vi "field emission sensor_v70.vi"() -> ()   [LabVIEW 2014]
uses:
  Keithley 24XX/Public/Data/Read (Single Point).vi
  Keithley 24XX/Keithley 24XX.lvlib
  <userlib>/Nanonis Prog Interface V5/Nanonis Prog Interface.lvlib
  <vilib>/Analysis/NI_AALBase.lvlib
panel:
  in  "Std threshold":dbl=5e-12 format="%#_6p"
  in  "Mean threshold":dbl=2e-11 format="%#_6p"
  out "ramp paused":bool
  out "x+y":sgl=1.4799449e-10
  out "amplitude":sgl(graph)=1.0739469e-11
  in  "Amplitude (V) (NaN=no change)":sgl=nan
  in  "Frequency (Hz) (NaN=no change)":sgl=nan format="%#_6p"
  in  "p Amplitude":dbl=-0.3 format="%#_6p"
  in  "amplitude max":sgl=1.5e-10 format="%#_6p"
  in  "Signal index (0-79)":i8=49
  out "amplitude":sgl=1.0739469e-11 format="%#_6p"
  in  "dz":dbl=1e-09 format="%#_6p"
  in  "ramp delay (s)":dbl=0.001
  out "ramp trigger":bool
  out "millisecond timer value":u32=272952714
  in  "Clear plots":bool
  out "z":dbl(graph)=7.783200430924225e-08
  in  "Ramp":bool
  in  "steps":sgl=5e-09 format="%#_6p"
  in  "Ramp to":sgl=1.3e-06 format="%#_6p"
  in  "I":sgl=5e-05 format="%#_6p"
  in  "PID":bool
  in  "p":sgl=0.01 format="%#_6p"
  in  "setpoint":sgl format="%#_3p"
  in  "max Current":sgl=2e-06 format="%#_6p"
  in  "setpoint approach":sgl=3e-08 format="%#_6p"
  in  "auto approach":bool
  in  "Number of steps":u16=1
  in  "withdraw tip":bool
  in  "coarse step":bool
  in  "Direction":enum16{"X +", "X -", "Y +", "Y -", "Z +", "Z -"}(ring)=enum."Z +"
  in  "Machine name (local machine IP)":string="localhost"
  in  "Z position [m]":dbl=7.783200430924225e-08 max=1.096e-07 step=1.0 format="%_6p"
  out "current [A]":sgl=-1.479945e-08 format="%#_6p"
  in  "time divider":dbl=60.0
  out "time elapsed":dbl=72.48559594154358
  in  "milliseconds to wait":u32=100
  in  "VISA resource name":refnum<visa-resource-name>="GPIB0::21::INSTR"
  in  "stop":bool
  in  "current multiplier":sgl=1.0
  out "Current":sgl(graph)=-1.479945e-08
  # "STOP the VI during an Nanonis Auto Approach"
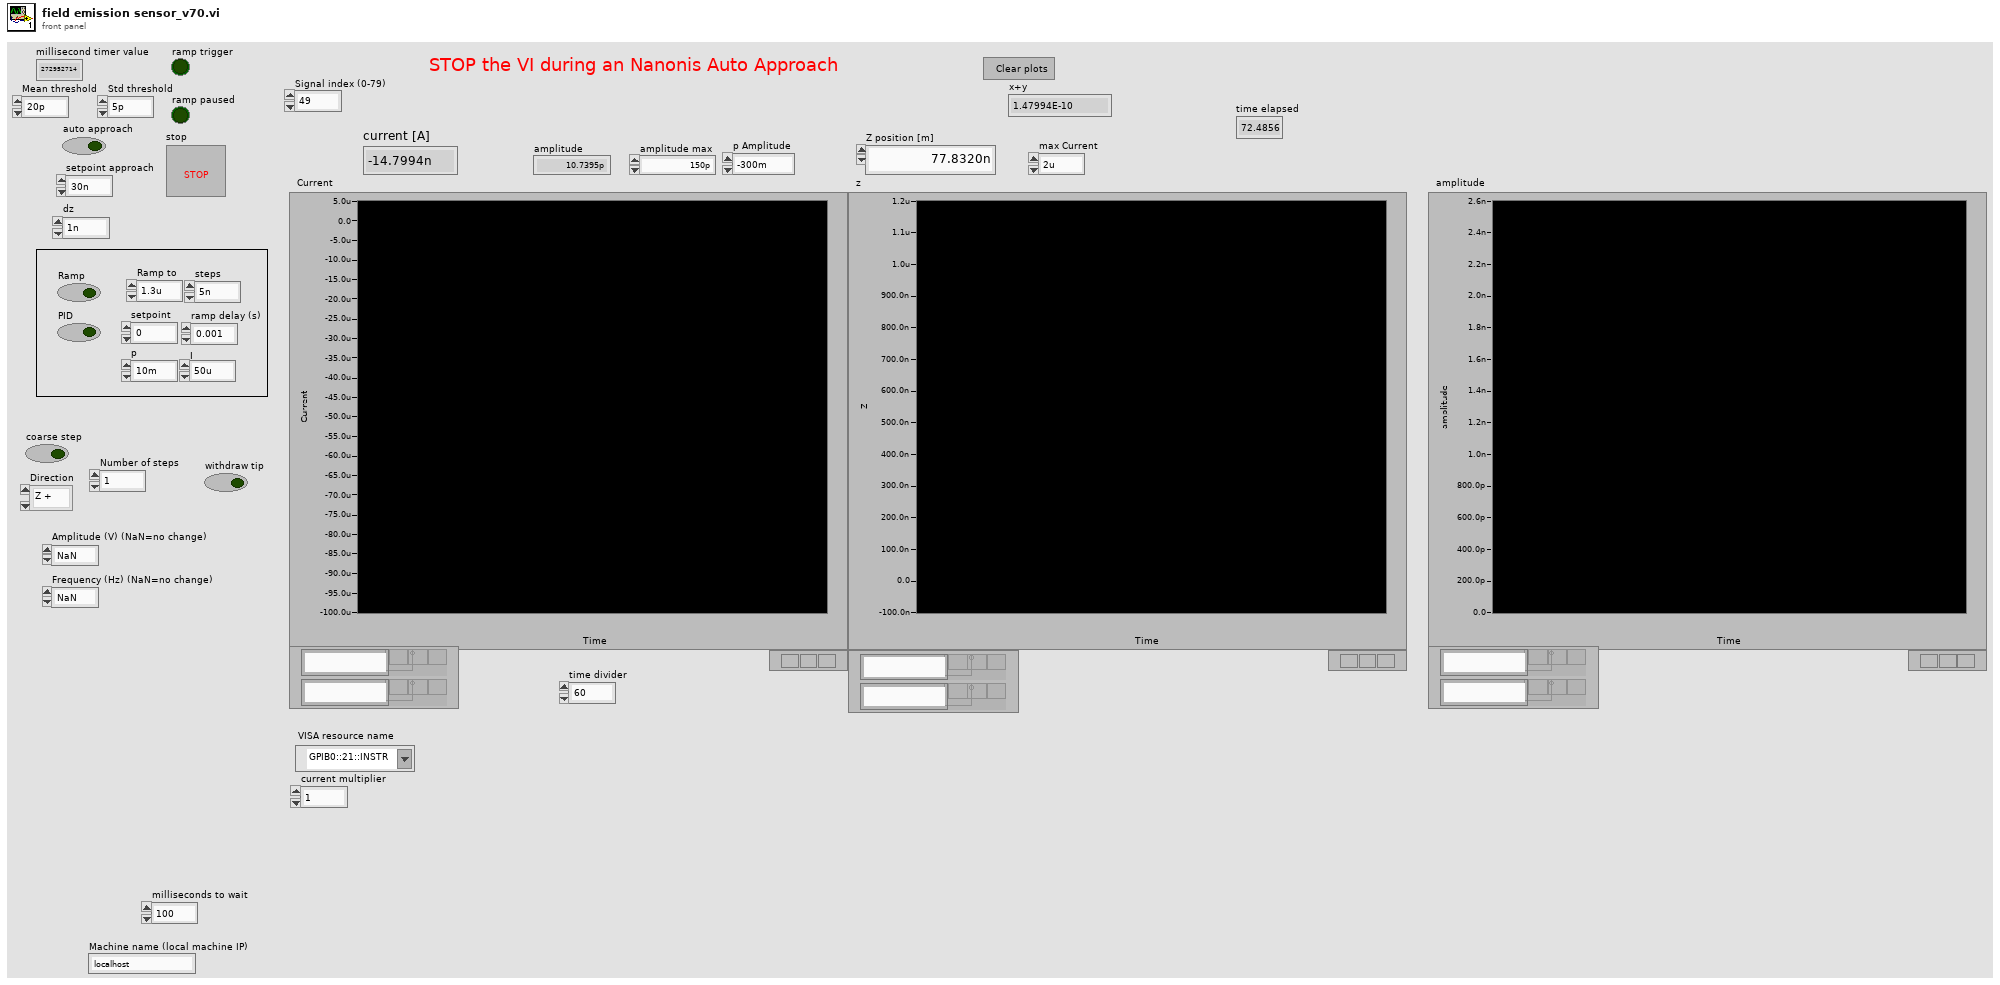
[diagram p1: front panel]
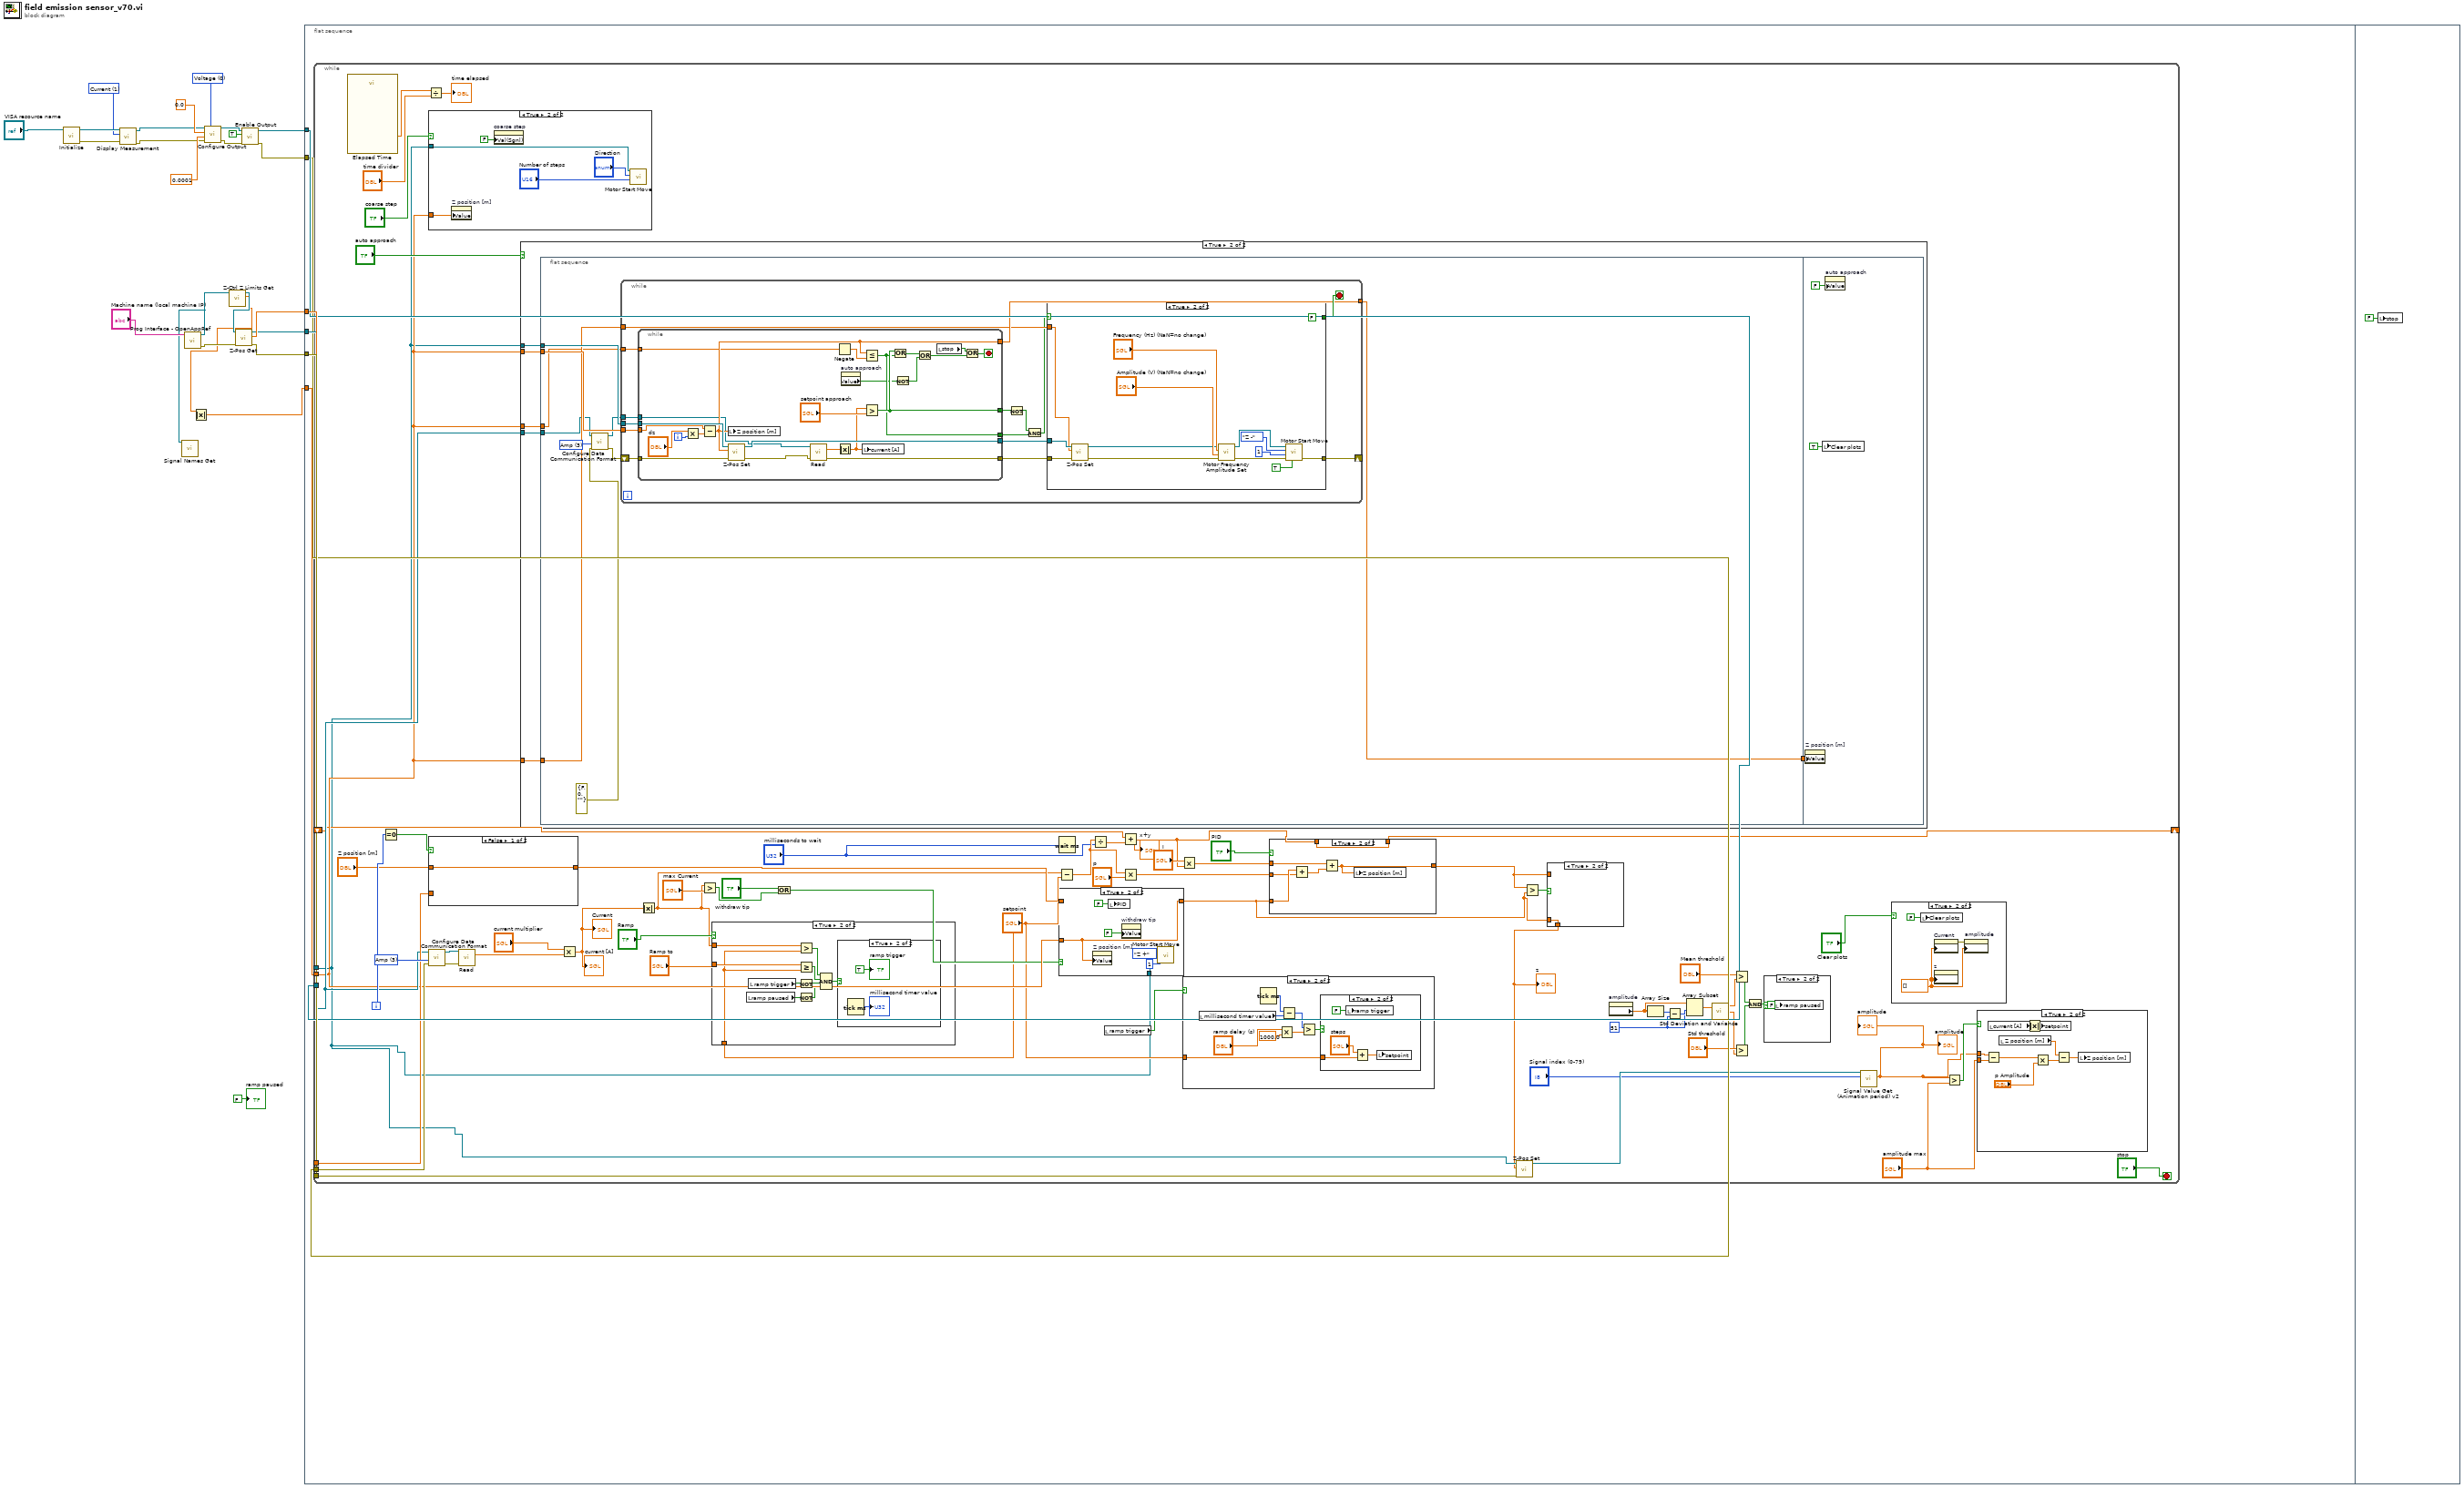
[diagram p0: block diagram]
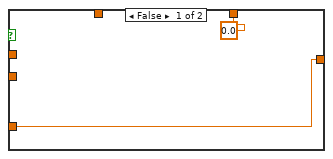
[diagram p10: hidden frame]
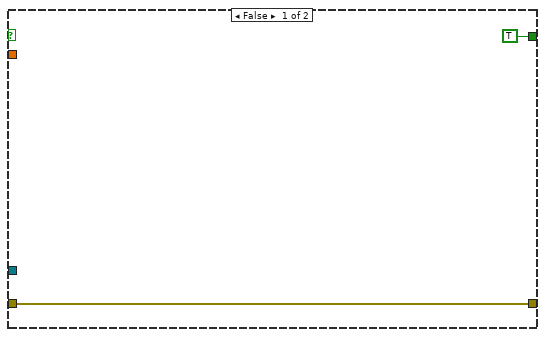
[diagram p12: hidden frame]
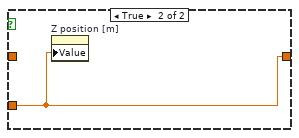
[diagram p15: hidden frame]
diagram:
  w6 = u16 1 items=["Voltage", "Current", "Resistance"] ("Displayed Measurement (0: Voltage)")
  w18 = u16 0 items=["Voltage", "Current"] ("Source Mode  (0: Voltage)")
  n1 = call "Initialize.vi"("VISA resource name"="VISA resource name") -> ("error out"=w8:errorcluster, "VISA resource name out"=w10:refnum<visa-resource-name>)  [unwired: 9 in]
  n2 = call "Display Measurement.vi"("error in (no error)"=w8, "Displayed Measurement (0: Voltage)"=w6, "VISA resource name"=w10) -> ("error out"=w7:errorcluster, "VISA resource name out"=w9:refnum<visa-resource-name>)  [unwired: 7 in]
  n3 = call <userlib>:"Prog Interface - OpenAppRef.vi"("Machine name (local machine IP)"="Machine name (local machine IP)") -> ("Error out"=w23:errorcluster, "Application reference"=w2:refnum<vi>)  [unwired: 5 in]
  n4 = call <userlib>:"Signal Names Get.vi"("Application ref in"=w2) -> ()  [unwired: 6 in, 3 out]
  n5 = call "Configure Output.vi"("Source Mode  (0: Voltage)"=w18, "error in (no error)"=w7, "Compliance  Level (0.1)"=0.0001, "Output Level (0)"=0.0, "VISA resource name"=w9) -> ("error out"=w14:errorcluster, "VISA resource name out"=w15:refnum<visa-resource-name>)  [unwired: 5 in]
  n6 = call <userlib>:"Z-Ctrl Z Limits Get.vi"("Application ref in"=w2) -> ("Z high limit"=w3:sgl, "Application ref out"=w4:refnum<vi>)  [unwired: 7 in, 2 out]
  n7 = Absolute Value(x=w3) -> (abs(x)=w5:sgl)
  n8 = call <userlib>:"Z-Pos Get.vi"("error in (no error)"=w23, "Application ref in"=w4) -> ("error out"=w22:errorcluster, "Z position (m)"=w21:sgl, "Application ref out"=w20:refnum<vi>)  [unwired: 7 in]
  n9 = call "Enable Output.vi"("error in (no error)"=w14, "Enable Output (T: Enable)"=TRUE, "VISA resource name"=w15) -> ("error out"=w11:errorcluster, "VISA resource name out"=w12:refnum<visa-resource-name>)  [unwired: 7 in]
  n10 = flat-sequence {
    tunnel: w22 -> [w30]
    tunnel: w21 -> [w29]
    tunnel: w20 -> [w28]
    tunnel: w12 -> [w27]
    tunnel: w11 -> [w26]
    tunnel: w5 -> [w25]
    frame #0 {
      n11 = while {
        tunnel: w28 -> [w47]
        tunnel: w30 -> [w86]
        tunnel: w29 -> [w85]
        tunnel: w27 -> [w77]
        tunnel: w26 -> [w76]
        tunnel: w25 -> [w74]
        shift-right: [w59] -> _
        shift-left: _ -> [w66]
        i -> [w84]
        stop <- "stop" stop-if-true
        w39 = 51 ("y")
        w90 = u16 3 items=["All", "Volt and Amp", "Volt", "Amp"] ("Data Selection (0: All)")
        n12 = call "Elapsed Time"() -> ("Elapsed Time (s)"=w87:dbl)  [unwired: 12 in, 7 out]
        n13 = Equal To 0?(x=w84) -> (x = 0?=w83:bool)
        n14 = Divide(x=w87, y="time divider") -> (x/y=→"time elapsed":dbl)
        n15 = case shown="True" "coarse step" {
          tunnel: w47 -> [_ w227]
          tunnel: w74 -> [_ w223]
          frame False {
          }
          frame True {
            n16 = property on="Z position [m]" class="DigNum (strict)"("Value"=w223) -> ()  [unwired: 2 in, 2 out]
            n17 = property on="coarse step" class="Bool (strict)"("Val(Sgnl)"=FALSE ("Value (Signaling)")) -> ()  [unwired: 2 in, 2 out]
            n18 = call <userlib>:"Motor Start Move.vi"("Number of steps"="Number of steps", "Direction"="Direction", "Application ref in"=w227) -> ()  [unwired: 6 in, 2 out]
          }
        }
        n19 = case shown="False" w83 {
          tunnel: [w228 w229] -> w80
          tunnel: w85 -> [_ w229]
          tunnel: "Z position [m]" -> [w228 _]
          frame False {
          }
          frame True {
            n20 = property on="Z position [m]" class="DigNum (strict)"("Value"=w229) -> ()  [unwired: 2 in, 2 out]
          }
        }
        n21 = call "Configure Data Communication Format.vi"("error in (no error)"=w76, "Data Selection (0: All)"=w90, "VISA resource name"=w77) -> ("error out"=w91:errorcluster, "VISA resource name out"=w92:refnum<visa-resource-name>)  [unwired: 7 in]
        n22 = call-poly "Read.vi"("VISA resource name"=w92, "error in (no error)"=w91) -> ("Current"=w94:sgl)  [unwired: 7 in, 6 out]
        n23 = case shown="True" "auto approach" {
          tunnel: w77 -> [_ w147]
          tunnel: w47 -> [_ w146]
          tunnel: w74 -> [_ w144]
          tunnel: w74 -> [_ w143]
          tunnel: w74 -> [_ w142]
          frame False {
          }
          frame True {
            n24 = flat-sequence {
              tunnel: w147 -> [w150]
              tunnel: w146 -> [w157]
              tunnel: [w156] -> w145
              tunnel: w144 -> [w155]
              tunnel: w143 -> [w154]
              tunnel: w142 -> [w153]
              tunnel: w145 -> [w214]
              frame #0 {
                w148 = u16 3 items=["All", "Volt and Amp", "Volt", "Amp"] ("Data Selection (0: All)")
                n25 = call "Configure Data Communication Format.vi"("error in (no error)"=errorcluster {"status"=FALSE, "code"=0, "source"=""}, "Data Selection (0: All)"=w148, "VISA resource name"=w150) -> ("error out"=w151:errorcluster, "VISA resource name out"=w149:refnum<visa-resource-name>)  [unwired: 7 in]
                n26 = while {
                  tunnel: w149 -> [w172]
                  tunnel: w157 -> [w171]
                  tunnel: [w165] -> w156
                  tunnel: w155 -> [w164]
                  tunnel: w154 -> [w163]
                  tunnel: w153 -> [w162]
                  shift-right: [w161] -> _
                  shift-left: w151 -> [w160]
                  stop <- w166 stop-if-true
                  n27 = while {
                    tunnel: w172 -> [w190]
                    tunnel: w171 -> [w210]
                    tunnel: [w209] -> w170
                    tunnel: [w208] -> w169
                    tunnel: [w207] -> w168
                    tunnel: [w192] -> w167
                    tunnel: [w206] -> w165
                    tunnel: w164 -> [w205]
                    tunnel: w162 -> [w203]
                    tunnel: w160 -> [w191]
                    i -> [w212]
                    stop <- w198 stop-if-true
                    n28 = Multiply(x="dz", y=w212) -> (x*y=w194:dbl)
                    n29 = Subtract(x=w205, y=w194) -> (x-y=w206:dbl)
                    n30 = local write "Z position [m]"(w206) -> ()
                    n31 = call <userlib>:"Z-Pos Set.vi"("error in (no error)"=w191, "Z position (m)"=w206, "Application ref in"=w210) -> ("error out"=w189:errorcluster, "Application ref out"=w207:refnum<vi>)  [unwired: 7 in]
                    n32 = call-poly "Read.vi"("VISA resource name"=w190, "error in (no error)"=w189) -> ("Current"=w211:sgl, "error out"=w192:errorcluster)  [unwired: 7 in, 5 out]
                    n33 = Negate(x=w203) -> (-x=w204:sgl)
                    n34 = Absolute Value(x=w211) -> (abs(x)=w195:sgl)
                    n35 = property on="auto approach" class="Bool (strict)"() -> ("Value"=w201:bool)  [unwired: 2 in, 2 out]
                    n36 = local write "current [A]"(w195) -> ()
                    n37 = Less Or Equal?(x=w206, y=w204) -> (x <= y?=w208:bool)
                    n38 = Greater?(x=w195, y="setpoint approach") -> (0:w209:bool)
                    n39 = Or(x=w209, y=w208) -> (x .or. y?=w202:bool)
                    n40 = Not(x=w201) -> (.not. x?=w200:bool)
                    n41 = Or(x=w202, y=w200) -> (x .or. y?=w199:bool)
                    n42 = local read "stop"() -> (w197:bool)
                    n43 = Or(x=w197, y=w199) -> (x .or. y?=w198:bool)
                  }
                  n44 = Not(x=w170) -> (.not. x?=w159:bool)
                  n45 = And(x=w159, y=w169) -> (x .and. y?=w158:bool)
                  n46 = case shown="True" w158 {
                    tunnel: w168 -> [_ w188]
                    tunnel: w167 -> [w173 w187]
                    tunnel: [TRUE FALSE] -> w166
                    tunnel: w163 -> [_ w183]
                    tunnel: [w173 w176] -> w161
                    frame False {
                    }
                    frame True {
                      n47 = call <userlib>:"Z-Pos Set.vi"("error in (no error)"=w187, "Z position (m)"=w183, "Application ref in"=w188) -> ("error out"=w180:errorcluster, "Application ref out"=w175:refnum<vi>)  [unwired: 7 in]
                      n48 = call <userlib>:"Motor Frequency Amplitude Set.vi"("Error in (no error)"=w180, "Amplitude (V) (NaN=no change)"="Amplitude (V) (NaN=no change)", "Frequency (Hz) (NaN=no change)"="Frequency (Hz) (NaN=no change)", "Application ref in"=w175) -> ("Error out"=w179:errorcluster, "Application ref out"=w181:refnum<vi>)  [unwired: 6 in]
                      n49 = call <userlib>:"Motor Start Move.vi"("Wait until finished? (F)"=TRUE, "Error in (no error)"=w179, "Number of steps"=u16 1, "Direction"=enum16{"X +", "X -", "Y +", "Y -", "Z +", "Z -"}."Z -", "Application ref in"=w181) -> ("Error out"=w176:errorcluster)  [unwired: 4 in, 1 out]
                    }
                  }
                }
              }
              frame #1 {
                n50 = property on="Z position [m]" class="DigNum (strict)"("Value"=w214) -> ()  [unwired: 2 in, 2 out]
                n51 = local write "Clear plots"(TRUE ("Clear plots")) -> ()
                n52 = property on="auto approach" class="Bool (strict)"("Value"=FALSE ("auto approach")) -> ()  [unwired: 2 in, 2 out]
              }
            }
          }
        }
        n53 = Multiply(x="current multiplier", y=w94) -> (x*y=w73:sgl)
        "Current" <- w73
        "current [A]" <- w73
        n54 = Absolute Value(x=w73) -> (abs(x)=w57:sgl)
        n55 = Greater?(x=w57, y="max Current") -> (0:w70:bool)
        n56 = case shown="True" "Ramp" {
          tunnel: w57 -> [_ w131]
          tunnel: "setpoint" -> [_ w128]
          tunnel: "Ramp to" -> [_ w129]
          frame False {
          }
          frame True {
            n57 = local read "ramp paused"() -> (w123:bool)
            n58 = local read "ramp trigger"() -> (w125:bool)
            n59 = Greater?(x=w131, y=w128) -> (0:w130:bool)
            n60 = Greater Or Equal?(x=w129, y=w128) -> (x >= y?=w126:bool)
            n61 = Not(x=w125) -> (.not. x?=w124:bool)
            n62 = Not(x=w123) -> (.not. x?=w122:bool)
            n63 = Compound Arithmetic op=AND(w130, w126, w124, w122) -> (w127:bool)
            n64 = case shown="True" w127 {
              frame False {
              }
              frame True {
                n65 = Tick Count (ms)() -> (millisecond timer value=→"millisecond timer value":u32)
                "ramp trigger" <- TRUE ("ramp")
              }
            }
          }
        }
        n66 = Or(x="withdraw tip", y=w70) -> (x .or. y?=w71:bool)
        n67 = Subtract(x=w57, y="setpoint") -> (x-y=w62:sgl)
        n68 = Wait (ms)(milliseconds to wait="milliseconds to wait") -> ()  [unwired: 1 out]
        n69 = case shown="True" w71 {
          tunnel: [w216 w221] -> w43
          tunnel: w80 -> [w216 _]
          tunnel: w74 -> [_ w221]
          tunnel: w47 -> [_ w219]
          frame False {
          }
          frame True {
            n70 = property on="Z position [m]" class="DigNum (strict)"("Value"=w221) -> ()  [unwired: 2 in, 2 out]
            n71 = local write "PID"(FALSE ("PID")) -> ()
            n72 = property on="withdraw tip" class="Bool (strict)"("Value"=FALSE ("withdraw tip")) -> ()  [unwired: 2 in, 2 out]
            n73 = call <userlib>:"Motor Start Move.vi"("Number of steps"=u16 1, "Direction"=enum16{"X +", "X -", "Y +", "Y -", "Z +", "Z -"}."Z +", "Application ref in"=w219) -> ()  [unwired: 6 in, 2 out]
          }
        }
        n74 = Divide(x=w62, y="milliseconds to wait") -> (x/y=w63:sgl)
        n75 = local read "ramp trigger"() -> (w53:bool)
        n76 = Add(x=w66, y=w63) -> (x+y=w60:sgl)
        "x+y" <- w60
        n77 = Multiply(x=w62, y="p") -> (x*y=w67:sgl)
        n78 = Multiply(x="I", y=w60) -> (x*y=w64:sgl)
        n79 = case shown="True" w53 {
          tunnel: "setpoint" -> [_ w110]
          frame False {
          }
          frame True {
            n80 = local read "millisecond timer value"() -> (w113:u32)
            n81 = Tick Count (ms)() -> (millisecond timer value=w114:u32)
            n82 = Multiply(x="ramp delay (s)", y=1000.0) -> (x*y=w107:dbl)
            n83 = Subtract(x=w114, y=w113) -> (x-y=w112:u32)
            n84 = Greater?(x=w112, y=w107) -> (0:w111:bool)
            n85 = case shown="True" w111 {
              tunnel: w110 -> [_ w116]
              frame False {
              }
              frame True {
                n86 = local write "ramp trigger"(FALSE ("ramp")) -> ()
                n87 = Add(x="steps", y=w116) -> (x+y=w118:sgl)
                n88 = local write "setpoint"(w118) -> ()
              }
            }
          }
        }
        n89 = case shown="True" "PID" {
          tunnel: w43 -> [w135 w141]
          tunnel: [w135 w137] -> w45
          tunnel: w67 -> [_ w140]
          tunnel: w64 -> [_ w138]
          tunnel: w60 -> [_ w136]
          tunnel: [sgl 0.0 w136] -> w59
          frame False {
          }
          frame True {
            n90 = Add(x=w141, y=w140) -> (x+y=w139:dbl)
            n91 = Add(x=w138, y=w139) -> (x+y=w137:dbl)
            n92 = local write "Z position [m]"(w137) -> ()
          }
        }
        n93 = Greater?(x=w45, y=w43) -> (0:w46:bool)
        n94 = case shown="True" w46 {
          tunnel: w45 -> [w96 _]
          tunnel: [w96 w97] -> w44
          tunnel: w43 -> [_ w97]
          frame False {
          }
          frame True {
          }
        }
        "z" <- w44
        n95 = call <userlib>:"Z-Pos Set.vi"("error in (no error)"=w86, "Z position (m)"=w44, "Application ref in"=w47) -> ("Application ref out"=w52:refnum<vi>)  [unwired: 7 in, 1 out]
        n96 = property on="amplitude" class="WFChart (strict)"() -> ("History Data"=w42:sgl[])  [unwired: 2 in, 2 out]
        n97 = Array Size(array=w42) -> (size(s)=w41:i32)
        n98 = Subtract(x=w41, y=w39) -> (x-y=w40:i32)
        n99 = Array Subset(array=w42, index=w40, length=w39) -> (w38:sgl[])
        n100 = call <vilib>:"Std Deviation and Variance.vi"("X"=w38) -> ("mean"=w37:dbl, "standard deviation"=w31:dbl)  [unwired: 1 in, 1 out]
        n101 = Greater?(x="Mean threshold", y=w37) -> (0:w33:bool)
        n102 = Greater?(x="Std threshold", y=w31) -> (0:w34:bool)
        n103 = And(x=w33, y=w34) -> (x .and. y?=w32:bool)
        n104 = case shown="True" w32 {
          frame False {
          }
          frame True {
            n105 = local write "ramp paused"(FALSE ("ramp paused")) -> ()
          }
        }
        n106 = call <userlib>:"Signal Value Get (Animation period) v2.vi"("Signal index (0-79)"="Signal index (0-79)", "Application ref in"=w52) -> ("Signal value"=w49:sgl)  [unwired: 6 in, 2 out]
        "amplitude" <- w49
        "amplitude" <- w49
        n107 = case shown="True" "Clear plots" {
          frame False {
          }
          frame True {
            w119 = dbl[] [] ("History Data")
            n108 = local write "Clear plots"(FALSE ("Clear plots")) -> ()
            n109 = property on="Current" class="WFChart (strict)"("History Data"=w119) -> (error out=w120:errorcluster)  [unwired: 2 in, 1 out]
            n110 = property on="z" class="WFChart (strict)"("History Data"=w119) -> ()  [unwired: 2 in, 2 out]
            n111 = property on="amplitude" class="WFChart (strict)"(error in=w120, "History Data"=w119) -> ()  [unwired: 1 in, 2 out]
          }
        }
        n112 = Greater?(x=w49, y="amplitude max") -> (0:w50:bool)
        n113 = case shown="True" w50 {
          tunnel: w49 -> [_ w104]
          tunnel: "amplitude max" -> [_ w103]
          frame False {
          }
          frame True {
            n114 = Subtract(x=w104, y=w103) -> (x-y=w102:sgl)
            n115 = local read "current [A]"() -> (w99:sgl)
            n116 = local read "Z position [m]"() -> (w106:dbl)
            n117 = Absolute Value(x=w99) -> (abs(x)=w98:sgl)
            n118 = Multiply(x=w102, y="p Amplitude") -> (x*y=w100:dbl)
            n119 = local write "setpoint"(w98) -> ()
            n120 = Subtract(x=w106, y=w100) -> (x-y=w105:dbl)
            n121 = local write "Z position [m]"(w105) -> ()
          }
        }
      }
    }
    frame #1 {
      n122 = local write "stop"(FALSE ("stop")) -> ()
    }
  }
  "ramp paused" <- FALSE ("ramp paused")
